vi "YOLO11_OBB_OpenVINO_img.vi"() -> ()   [LabVIEW 2018]
doc: "YOLO11_OBB_OpenVINO_img: This example demonstrates object detection with oriented bounding boxes (OBB) using the YOLOv8 algorithm for image processing with OpenVINO. The example uses the YOLO11 model to detect objects in an image and outputs oriented bounding boxes (OBB) that accurately represent the position and rotation of each object. This approach allows for detecting objects that may not align with the traditional axis-aligned bounding boxes, making it suitable for applications such as detecting rotated objects, road signs, or irregularly shaped items in images. The integration with OpenVINO ensures optimized inference performance, enabling real-time processing on various hardware platforms."
uses:
  vi.lib/VIRobotics/ModelZoo/Object_Detection/yolov8_obb_openvino/Initial_yolov8_Obb_OpenVINO.vi
  vi.lib/VIRobotics/ModelZoo/Object_Detection/yolov8_obb_openvino/yolov8_obb_openvino.lvclass
  vi.lib/VIRobotics/opencv_yiku/Mat/Mat_8U/Mat_8U.lvclass
  vi.lib/VIRobotics/opencv_yiku/opencv_yiku.lvlib
panel:
  in  "pic_path":path=path "C:/ProgramData/VIRobotics/ModelZoo/Object_Detection/imgs/test.png"
  in  "device_name":string(combo)="CPU"
  in  "class_names_file":path=path "C:/ProgramData/VIRobotics/ModelZoo/Object_Detection/coco.names"
  in  "model_file":path=path "C:/ProgramData/VIRobotics/ModelZoo/Object_Detection/yolo11_obb/onnx_model/yolo11n-obb.onnx"
  out "picture":picture
  # "Overview: Demonstrates how to use the VIRobotics OpenVINO toolkit to load the the ONNX model of yolo11_obb for real-time object detection.\nRequirements: Windows.\nInstructions: \n1.Select the device_name to use.（If your computer has Intel GPU, you can select GPU in the \"type\" control before running the VI to achieve faster inference).\n2.Run the VI.\nIf you want to load the model you trained, follow the following steps:\n1.Select the device_name to use. \n2.Specify the model_file and class_names_file.\n3.Run the VI."
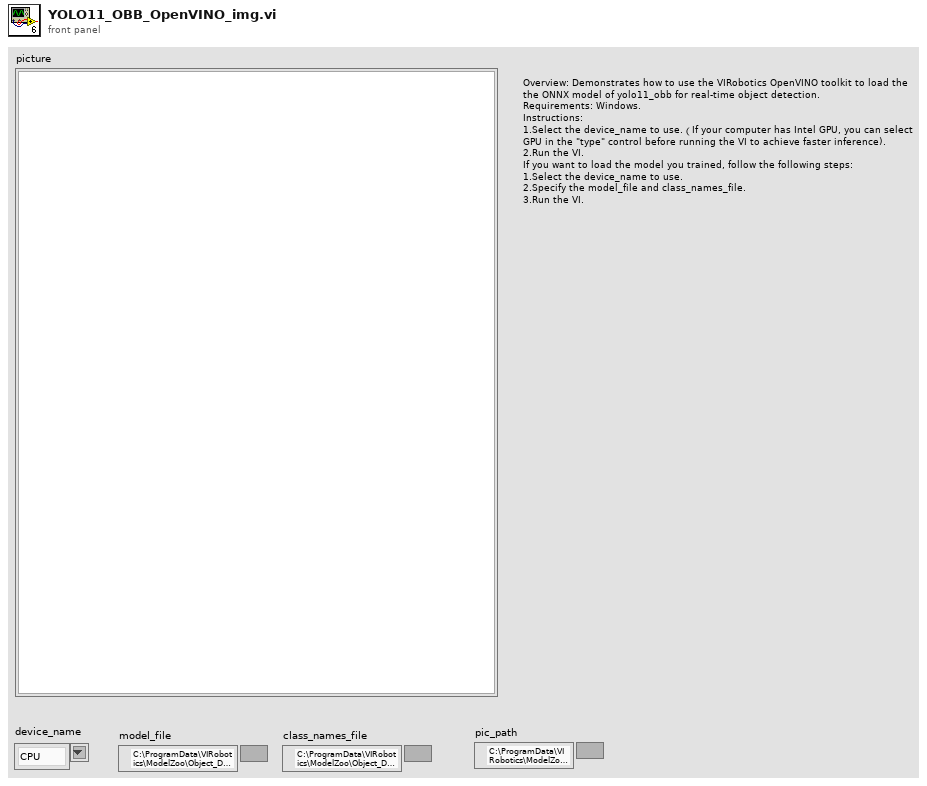
[diagram p1: front panel]
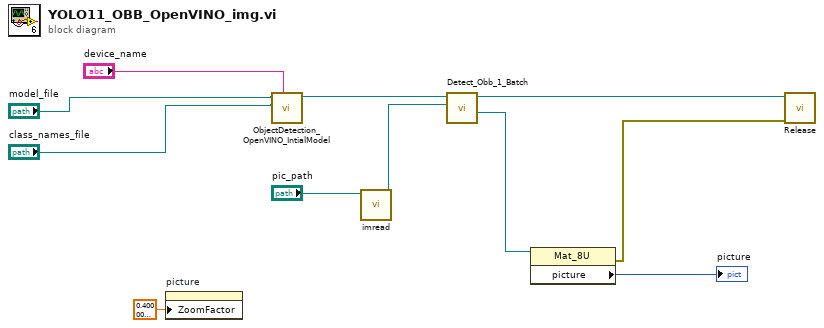
[diagram p0: block diagram]
diagram:
  n1 = property on="picture" class="Pict"("ZoomFactor"=sgl 0.4 ("Zoom Factor")) -> ()  [unwired: 2 in, 2 out]
  n2 = call-poly "ObjectDetection_OpenVINO_IntialModel.vi"("device_name"="device_name", "class_names_path"="class_names_file", "path"="model_file") -> ("yolov8_obb_ov out"=w4:refnum<class "yolov8_obb_openvino.lvclass">)  [unwired: 7 in, 1 out]
  n3 = call "imread.vi"("path"="pic_path") -> ("Mat out"=w10:refnum<class "Mat_8U.lvclass">)  [unwired: 9 in, 1 out]
  n4 = call-dynamic "Detect_Obb_1_Batch.vi"("image"=w10, "yolov8_obb_openvino in"=w4) -> ("image out"=w9:refnum<class "Mat_8U.lvclass">, "yolov8_obb_openvino out"=w11:refnum<class "yolov8_obb_openvino.lvclass">)  [unwired: 6 in, 2 out]
  n5 = property class="Mat_8U"(reference=w9) -> (error out=w8:errorcluster, "picture"=→"picture":picture)  [unwired: 1 in, 1 out]
  n6 = call-dynamic "Release.vi"("error in (no error)"=w8, "yolov8_obb_openvino in"=w11) -> ()  [unwired: 8 in, 2 out]
